vi "EnableDisable - Right Click.vi"(8 "error in (no error)":errorcluster, 11 "Node Ptr":u64 format="%.0x") -> (0 "error out":errorcluster)   [LabVIEW 2019, in "Ballard Arinc-429 System Explorer.lvlib"]
uses:
  Ballard Arinc-429 System Explorer.lvlib
  Shared/Controls and Global/Global.vi
  <vilib>/NI VeriStand/Custom Device API/Custom Device API.lvlib
  Shared/Ballard Arinc-429 Shared.lvlib
panel:
  in  "Tag":string
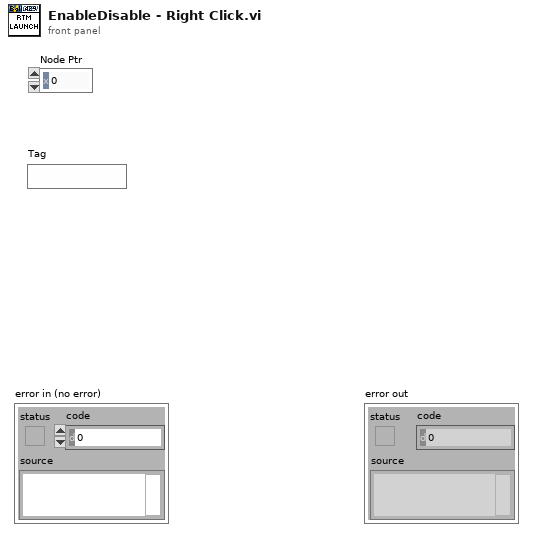
[diagram p1: front panel]
types:
  T1 = typedef "Custom Device API.lvlib/Custom Device Item Ref.ctl" = u64
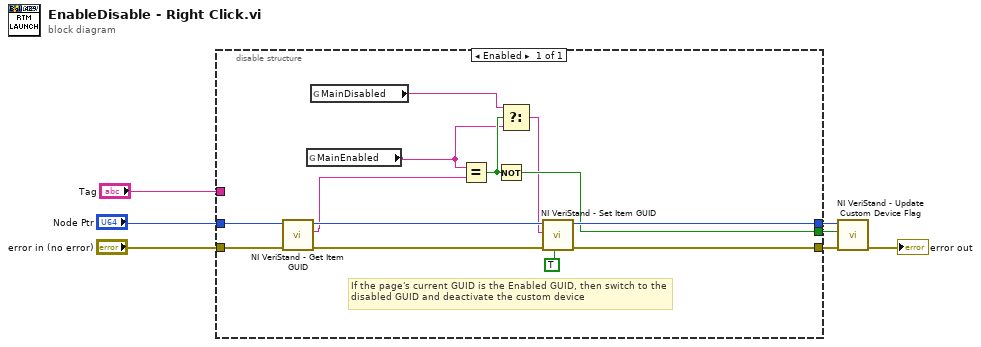
[diagram p0: block diagram]
diagram:
  n1 = disable-structure shown="Enabled" {
    disable-tunnel: [w10] -> w7
    disable-tunnel: [w17] -> w6
    disable-tunnel: [w16] -> w5
    disable-tunnel: "Node Ptr" -> [w15]
    disable-tunnel: "error in (no error)" -> [w14]
    disable-tunnel: "Tag" -> [_]
    frame Enabled {
      # "If the page's current GUID is the Enabled GUID, then switch to the disabled GUID and deactivate the custom device"
      n2 = call <vilib>:"NI VeriStand - Get Item GUID.vi"("error in (no error)"=w14, "Item Ref in"=w15) -> ("error out"=w19:errorcluster, "GUID"=w9:string, "Item Ref out"=w18:T1)  [unwired: 7 in]
      n3 = global read "Global.vi" "MainEnabled"() -> (w11:string)
      n4 = global read "Global.vi" "MainDisabled"() -> (w12:string)
      n5 = Equal?(x=w11, y=w9) -> (x = y?=w13:bool)
      n6 = Not(x=w13) -> (.not. x?=w16:bool)
      n7 = Select(t=w12, s=w13, f=w11) -> (s? t:f=w8:string)
      n8 = call <vilib>:"NI VeriStand - Set Item GUID.vi"("Refresh System Explorer Tree? (F)"=TRUE, "error in (no error)"=w19, "GUID"=w8, "Item Ref in"=w18) -> ("error out"=w10:errorcluster, "Item Ref out"=w17:T1)  [unwired: 6 in]
    }
  }
  n9 = call <vilib>:"NI VeriStand - Update Custom Device Flag.vi"("error in (no error)"=w7, "Is Custom Device Active?"=w5, "Device Ref in"=w6) -> ("error out"=→"error out":errorcluster)  [unwired: 7 in, 1 out]
